vi "addUnmarkedSum.vi"(10 "Numeric":i32, 11 "BingoBoard in":refnum<class "BingoBoard.lvclass">) -> (3 "output cluster":refnum<class "BingoBoard.lvclass">)   [LabVIEW 2017, in "BingoBoard.lvclass"]
uses:
  BingoBoard.lvclass
  BingoBoard.lvclass/BingoBoard.ctl
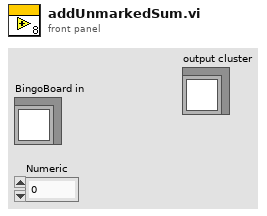
[diagram p1: front panel]
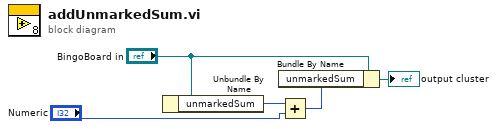
[diagram p0: block diagram]
diagram:
  n1 = Unbundle By Name("BingoBoard in") -> ("unmarkedSum"=w2:i32)
  n2 = Add(x=w2, y="Numeric") -> (x+y=w5:i32)
  n3 = Bundle By Name(cluster="BingoBoard in", "unmarkedSum"=w5) -> (→"output cluster":refnum<class "BingoBoard.lvclass">)
